vi "Handle mouse leave.vi"(8 "error in (no error)":errorcluster, 11 "Bool D Element in":refnum<class "Bool D Element.lvclass">) -> (0 "error out":errorcluster, 3 "Bool D Element out":refnum<class "Bool D Element.lvclass">)   [LabVIEW 2020, in "D Datagrid Library.lvlib" / "Bool D Element.lvclass"]
uses:
  Bool D Element.lvclass
  Bool D Element.lvclass/Bool D Element.ctl
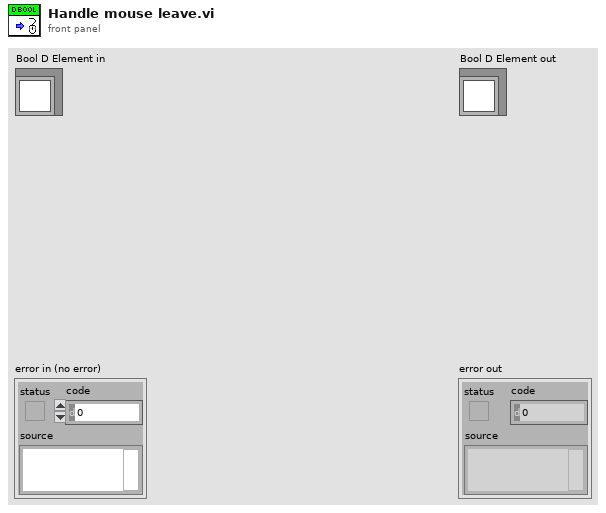
[diagram p1: front panel]
types:
  T1 = typedef "LVFontTypeDef.ctl" = cluster{"Font Name":string, "Size":u16, "Bold":bool, "Italic":bool, "Underline":bool, "Strikeout":bool, "Color":u32}
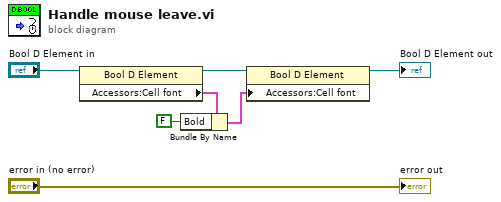
[diagram p0: block diagram]
diagram:
  n1 = property class="Bool D Element"(reference="Bool D Element in") -> (reference out=w6:refnum<class "Bool D Element.lvclass">, "Accessors:Cell font"=w5:T1)  [unwired: 1 in, 1 out]
  n2 = Bundle By Name(cluster=w5, "Bold"=FALSE) -> (w4:T1)
  n3 = property class="Bool D Element"(reference=w6, "Accessors:Cell font"=w4) -> (reference out=→"Bool D Element out":refnum<class "Bool D Element.lvclass">)  [unwired: 1 in, 1 out]
  "error out" <- "error in (no error)"
